vi "AudioConfig_OBJ.vi"(7 "Mode":enum16{"Get", "Set"}(ring), 8 "error in":errorcluster, 11 "PROPERTIES IN":T1={"Speaker Device ID"=0, "Microphone Device ID"=0, "sound format"={"sample rate (S/s)"=32000.0, "number of channels"=1, "bits per sample"=16}, "number of samples/ch"=8280}) -> (0 "error out":errorcluster, 3 "PROPERTIES OUT":T1={"Speaker Device ID"=128, "Microphone Device ID"=0, "sound format"={"sample rate (S/s)"=32000.0, "number of channels"=1, "bits per sample"=16}, "number of samples/ch"=8280})   [LabVIEW 2013]
uses:
  AudioConfig_OBJ - PROP.ctl
  <vilib>/sound2/lvsound2.llb/Sound Data Format.ctl
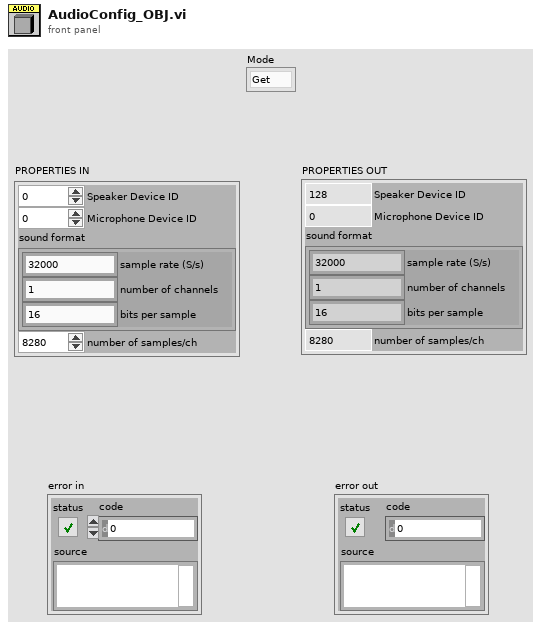
[diagram p1: front panel]
types:
  T1 = typedef "AudioConfig_OBJ - PROP.ctl" = cluster{"Speaker Device ID":u32, "Microphone Device ID":u32, "sound format":T2, "number of samples/ch":i32}
  T2 = typedef "Sound Data Format.ctl" = cluster{"sample rate (S/s)":dbl, "number of channels":i32, "bits per sample":i32}
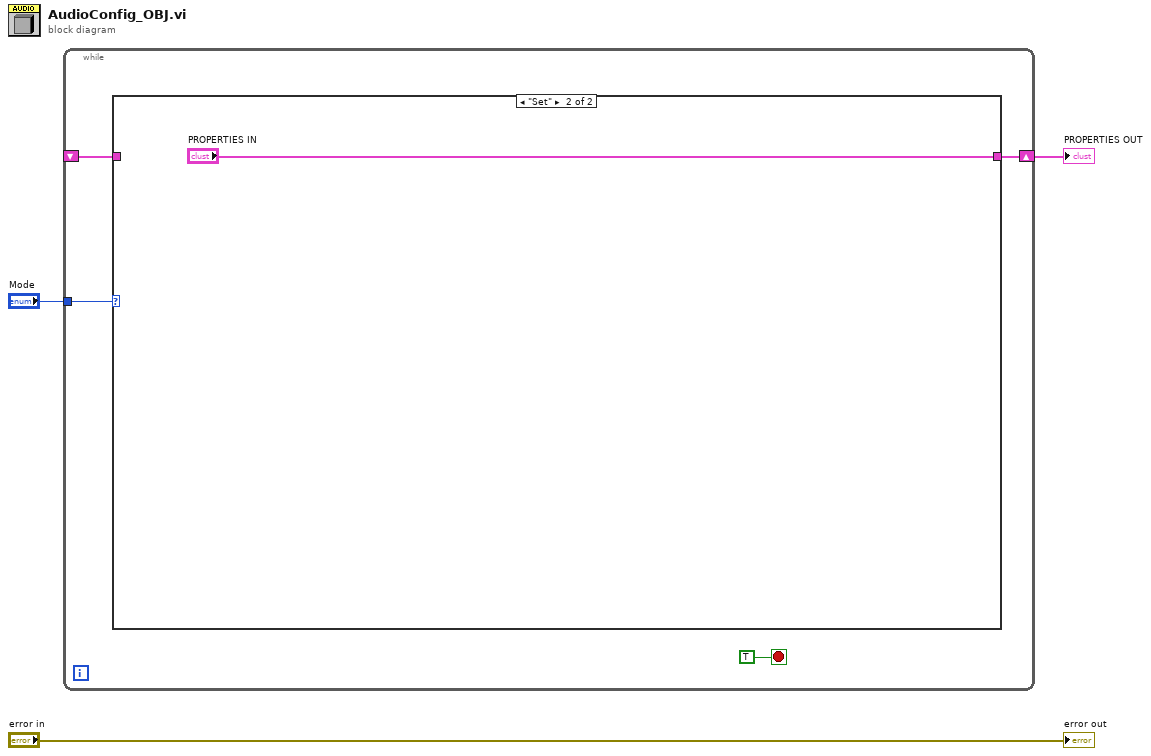
[diagram p0: block diagram]
diagram:
  n1 = while {
    tunnel: "Mode" -> [w6]
    shift-right: [w5] -> w2
    shift-left: _ -> [w4]
    stop <- TRUE stop-if-true
    n2 = case shown="\"Set\"" w6 {
      tunnel: [w8 "PROPERTIES IN"] -> w5
      tunnel: w4 -> [w8 _]
      frame "Get", Default {
      }
      frame "Set" {
      }
    }
  }
  "PROPERTIES OUT" <- w2
  "error out" <- "error in"
